vi "H-MEDI HardWareCtl.vi"() -> ()   [LabVIEW 2023]
uses:
  Controller/commonBtn.ctl
  <vilib>/Platform/TimedLoop/XDataNode/timing_clust.ctl
  <vilib>/Platform/TimedLoop/XDataNode/nitl_modes.ctl
  <vilib>/Platform/TimedLoop/XDataNode/wakeup.ctl
  <vilib>/Utility/miscctls.llb/LVPointTypeDef.ctl
  globalValue.vi
  <vilib>/Platform/TimedLoop/XDataNode/XDataNode.xnode
  <vilib>/Platform/TimedLoop/XDataNode/XDNodeRunTimeDep.lvlib
panel:
  in  "정지":bool
  out "userHeight":string
  out "userAge":string
  out "userGender":string
  in  "보행정보Menu":bool
  out "Tab":enum32{"1", "2", "3", "4", "Set"}(tab)
  out "rightIndicator#1-1":dbl
  out "leftIndicator#1-1":dbl
  out "leftIndicator#2-1":dbl
  out "rightIndicator#2-1":dbl
  out "leftIndicator#2-2":dbl
  out "rightIndicator#2-2":dbl
  out "leftIndicator#3-1":dbl
  out "rightIndicator#3-1":dbl
  out "leftIndicator#3-2":dbl
  out "rightIndicator#3-2":dbl
  out "leftIndicator#3-3":dbl
  out "rightIndicator#3-3":dbl
  out "leftIndicator#4-1":dbl
  out "rightIndicator#4-1":dbl
  out "leftIndicator#4-2":dbl
  out "rightIndicator#4-2":dbl
  out "leftIndicator#4-3":dbl
  out "rightIndicator#4-3":dbl
  out "leftIndicator#4-4":dbl
  out "rightIndicator#4-4":dbl
  in  "monitoringDataSet":bool
  in  "보행 지표":T1
  in  "Home":bool
  out "userInfo":string="000cm /  00kg"
  out "roleInfo":string
  out "R_GCP":dbl(slide) scale=0.0..100.0
  out "L_GCP":dbl(slide) scale=0.0..100.0
  out "R_THIGH":sgl
  out "L_Force":sgl
  out "R_Force":sgl
  out "Ref_L":sgl
  out "Ref_R":sgl
  out "Velocity_L":sgl
  out "Pos_L":sgl
  out "Velocity_R":sgl
  out "Pos_R":sgl
  out "L_THIGH":sgl
  in  "System Off":bool
  in  "start":bool
  in  "stop":bool
  in  "tabButton":enum32{"기본설정", "세부 설정", "메모"}(radio)
  out "Time":dbl format="%<%H:%M:%S>t"
  out "담당자 이름":string caption="담당자:"
  out "userName":string
  in  "Error":bool
  out "Battery":u16(ring)
  in  "Bluetooth":bool
  in  "사이드 탭":enum32{"Total", "Right", "Left", "메모"}(tab)
  in  "totalUserContolForce":T2
  in  "totalUserContolRelease":T2
  in  "totalUserContolPeak":T2
  in  "totalUserContolOnset":T2
  in  "leftUserContolRelease":T2
  in  "leftUserContolOnset":T2
  in  "leftUserContolPeak":T2
  in  "leftUserContolForce":T2
  in  "rightUserContolPeak":T2
  in  "rightUserContolOnset":T2
  in  "rightUserContolRelease":T2
  in  "rightUserContolForce":T2
  in  "메모 컨트롤":string="메모를 입력하세요."
  in  "메모 설정":bool
  out "Exit?":bool=TRUE
  in  "Connect":bool
  in  "Setting Value":T3={"Output High"=40.0, "Output Low"=-40.0, "Vel_FindBase"=5.0, "Ref.Load_FindBase"=5.0, "Force Peak"=0.0, "L_기준값"=81.0, "L_검출값"=103.0, "L_End%"=39.0, "L_Peak%"=25.0, "L_Onset%"=0.0, "L_Pos"=0.0, "L_Offset"=0.0, "R_기준값"=81.0, "R_검출값"=103.0, "R_End%"=39.0, "R_Peak%"=25.0, "R_Onset%"=0.0, "R_Pos"=0.0, "R_Offset"=0.0}
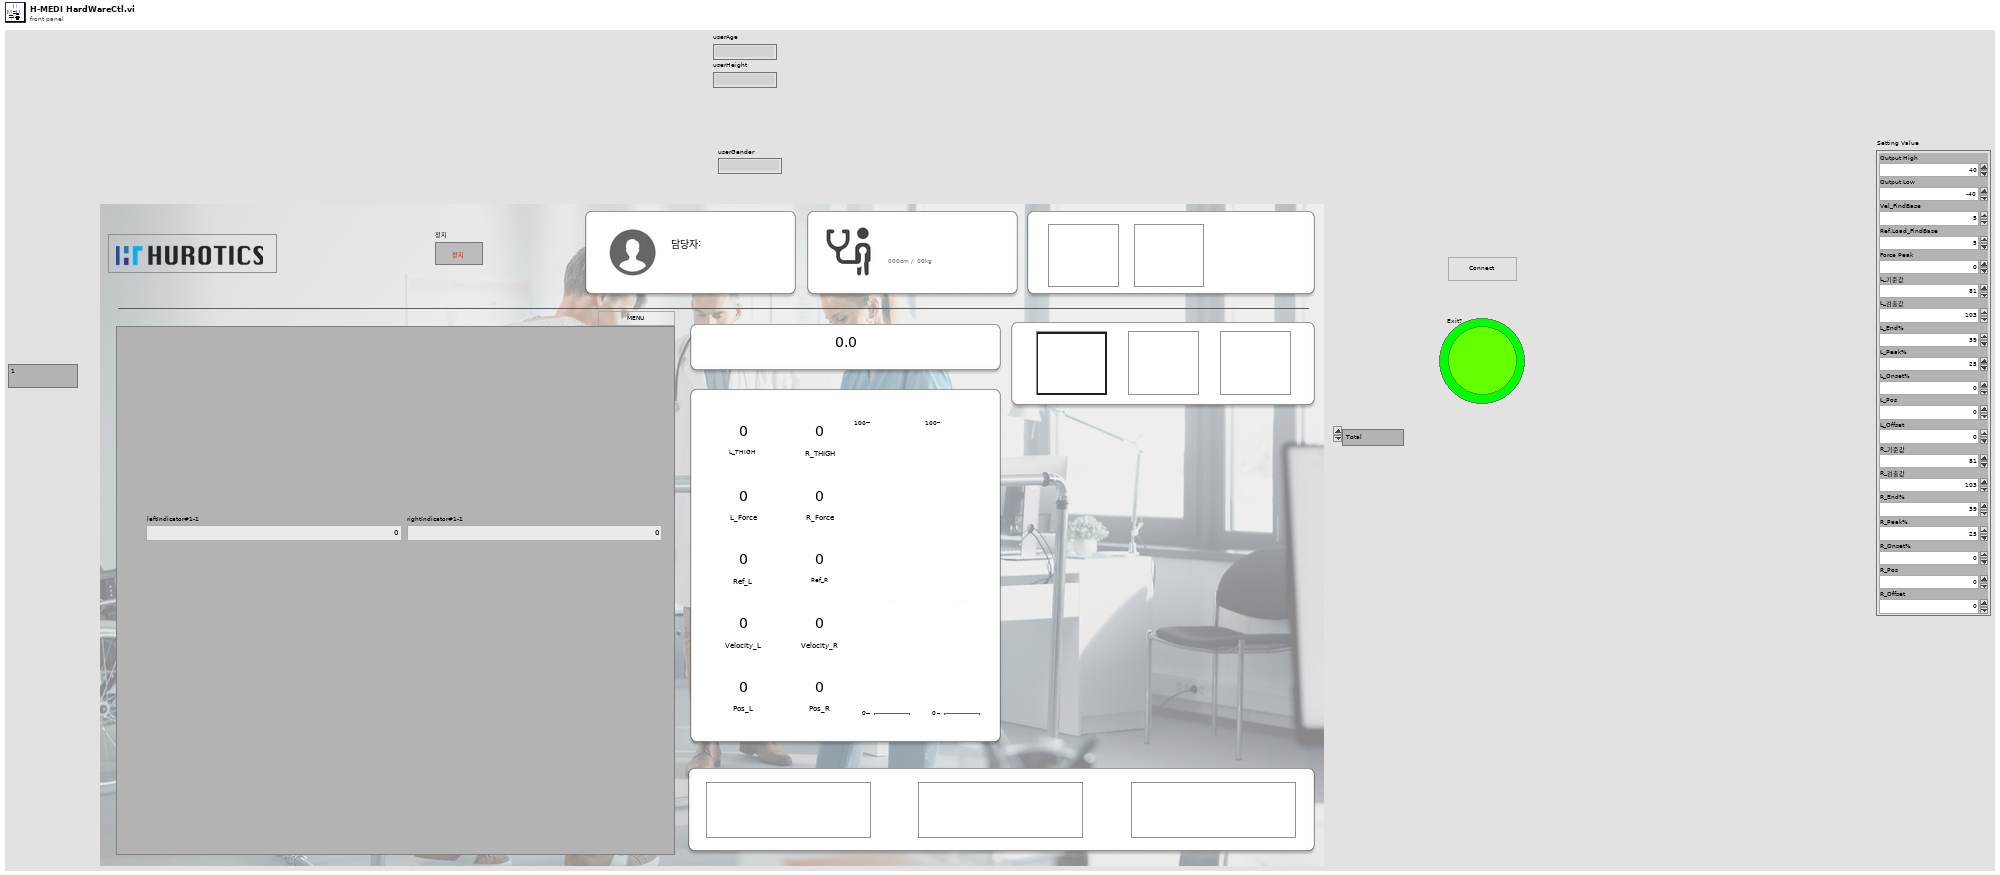
[diagram p1: front panel]
types:
  T1 = cluster{"고관절 각도":bool, "보행 속도":bool, "보행 거리":bool, "분당 걸음 수":bool, "보폭":bool, "Flexion / Extention":bool, "Range of Motion (ROM)":bool, "현 신체 균형":bool, "좌측만 보기":bool, "우측만 보기":bool}
  T2 = typedef "commonBtn.ctl" = i32
  T3 = cluster{"Output High":sgl, "Output Low":sgl, "Vel_FindBase":sgl, "Ref.Load_FindBase":sgl, "Force Peak":sgl, "L_기준값":sgl, "L_검출값":sgl, "L_End%":sgl, "L_Peak%":sgl, "L_Onset%":sgl, "L_Pos":sgl, "L_Offset":sgl, "R_기준값":sgl, "R_검출값":sgl, "R_End%":sgl, "R_Peak%":sgl, "R_Onset%":sgl, "R_Pos":sgl, "R_Offset":sgl}
  T4 = typedef "LVPointTypeDef.ctl" = cluster{"Horizontal":i16, "Vertical":i16}
  T5 = enum16{"connection", "create", "getReadList", "getRead", "getCount", "update", "delete", "close"}
  T6 = cluster{"baud rate (9600)":u32, "flow control (0:none)":u16, "VISA resource name 2":refnum<visa-resource-name>, "termination char\n(0xA = '\\n' = LF) ":u8, "data bits (8)":u16, "parity (0:none)":enum16{"None", "Odd", "Even", "Mark", "Space"}, "timeout (10sec)":u32, "Enable Termination\nChar (T)":bool, "stop bits (10: 1 bit)":u16}
  T7 = typedef "XDNodeRunTimeDep.lvlib/timing_clust.ctl" = cluster{"Expected End [f-1]":u64, "Actual End [f-1]":u64, "Finished Late? [f-1]":bool, "Expected End [i-1]":u64, "Actual End [i-1]":u64, "Finished Late? [i-1]":bool, "Expected Start [i]":u64, "Actual Start [i]":u64, "Expected Start [f]":u64, "Actual Start [f]":u64, "Source Name":string, "Structure Name":string, "Period":i64, "Deadline":i64, "Offset":i64, "Start":i64, "Priority":i32, "Timeout":i32, "Mode":T8, "Wakeup Reason":T9, "Error":errorcluster, "Source Type":string, "Secondary Source Type":string, "Global End Time":u64, "Global Start Time":u64, "Frame Duration":u64, "Iteration Duration":u64, "Assigned CPU":i32, "I/O Scan Engine Mode":u32}
  T8 = typedef "XDNodeRunTimeDep.lvlib/nitl_modes.ctl" = enum32{"No Change", "Process missed periods, maintain original phase", "Discard missed periods, maintain original phase", "Process missed periods, ignore original phase", "Discard missed periods, ignore original phase"}
  T9 = typedef "XDNodeRunTimeDep.lvlib/wakeup.ctl" = enum32{"Normal", "Aborted", "Asynchronous wakeup", "Timing source error", "Timed loop error", "Timeout"}
  T10 = enum16{"Open", "Write Only", "Read Only", "Write&Read", "Close"}
  T11 = enum16{"Init", "LogIn", "SignUpView", "Home", "Management_patientList", "Management_patientTrashtList", "Management_patientCreate", "Management_patientUpdate", "Management_patientTraining", "Management_patientTrainingDetail", "H-MEDI PatientList", "H-MEDI HardwareCtl", "Adjust", "FineTuning", "UserList", "UserDetail", "Exit"}
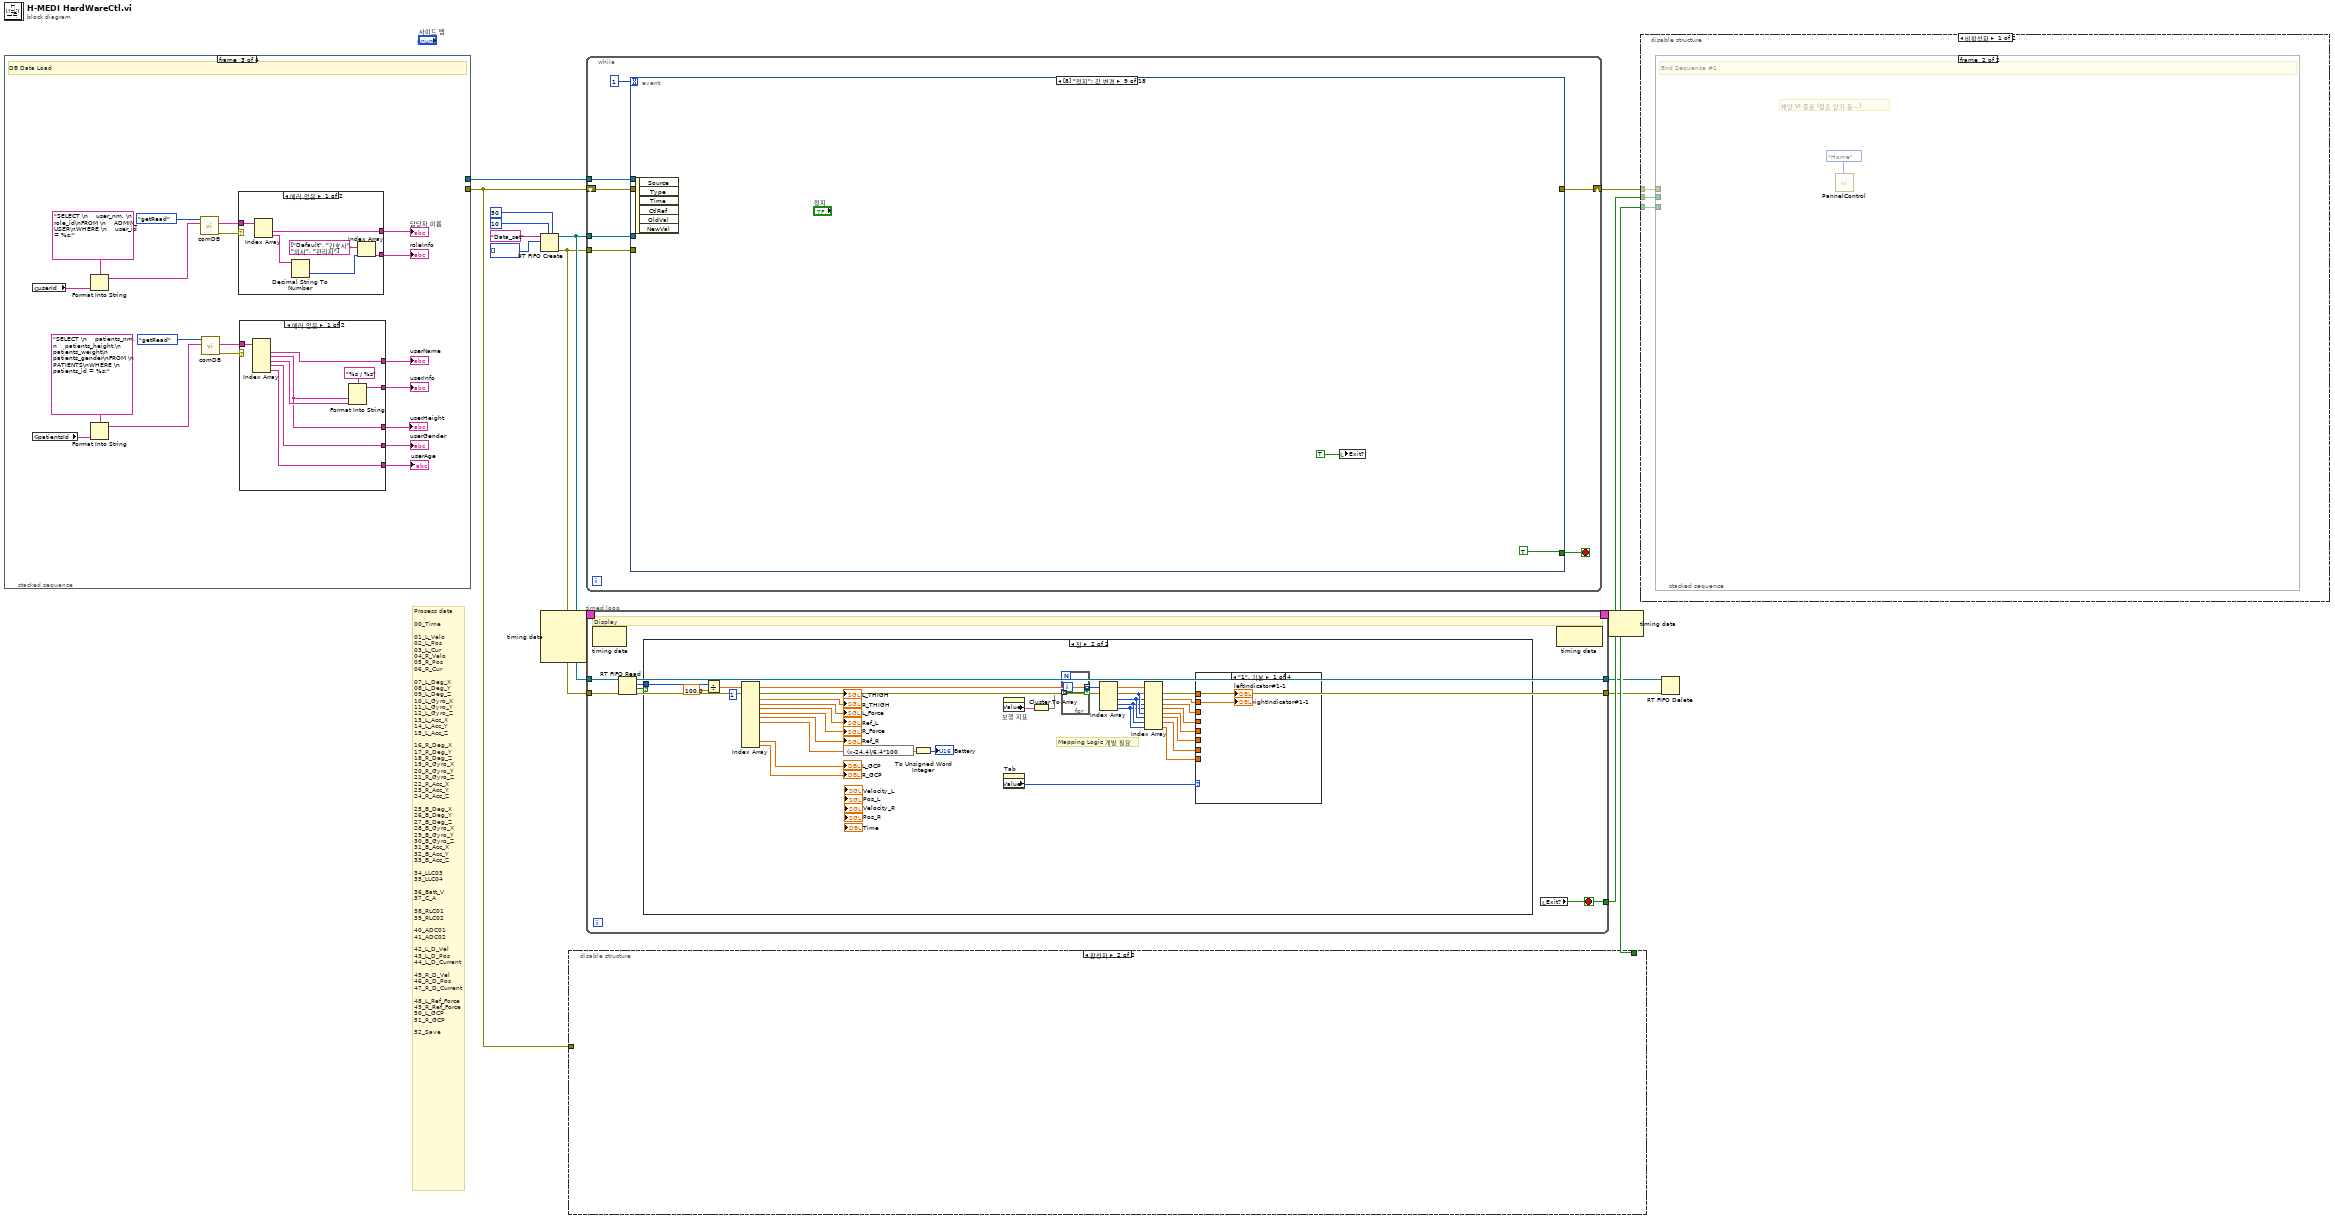
[diagram p0: block diagram]
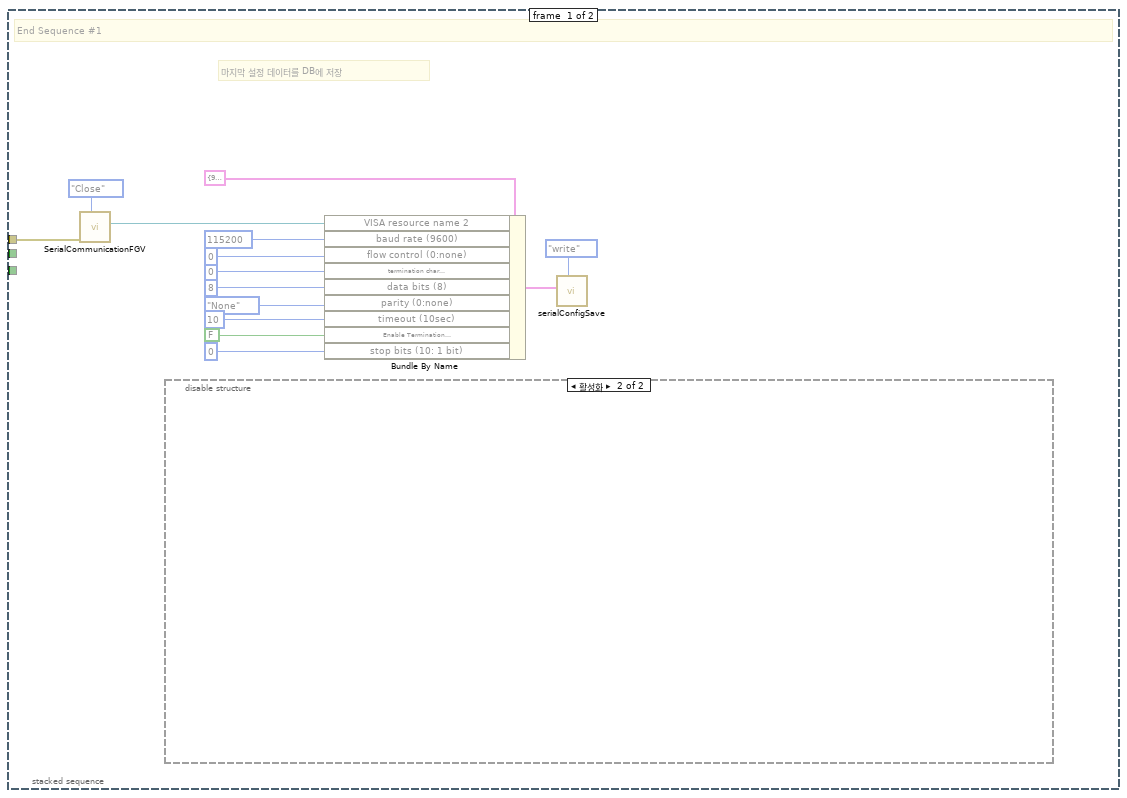
[diagram p2: hidden frame]
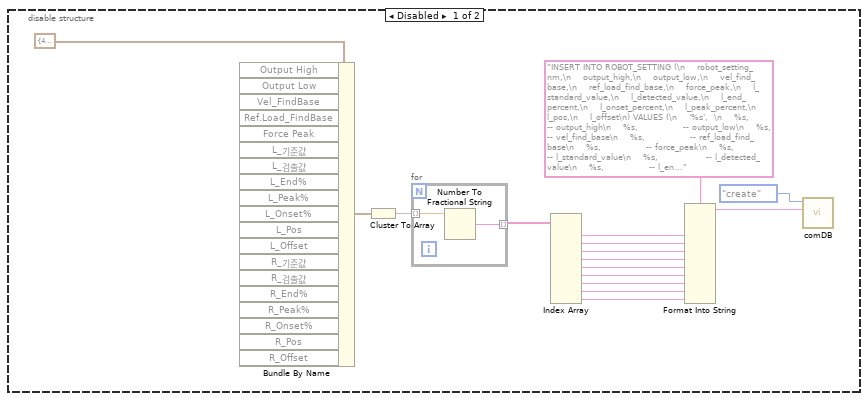
[diagram p3: hidden frame]
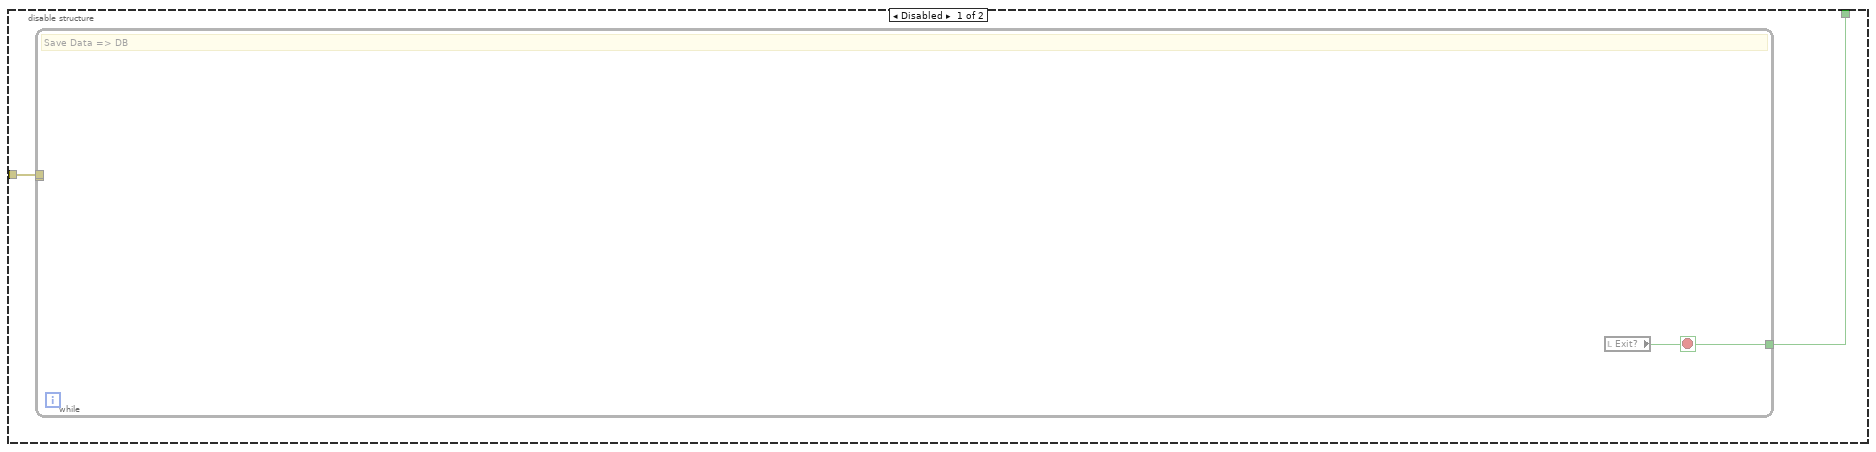
[diagram p5: hidden frame]
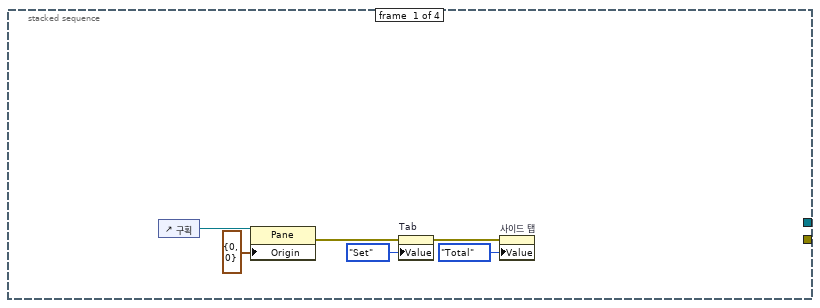
[diagram p6: hidden frame]
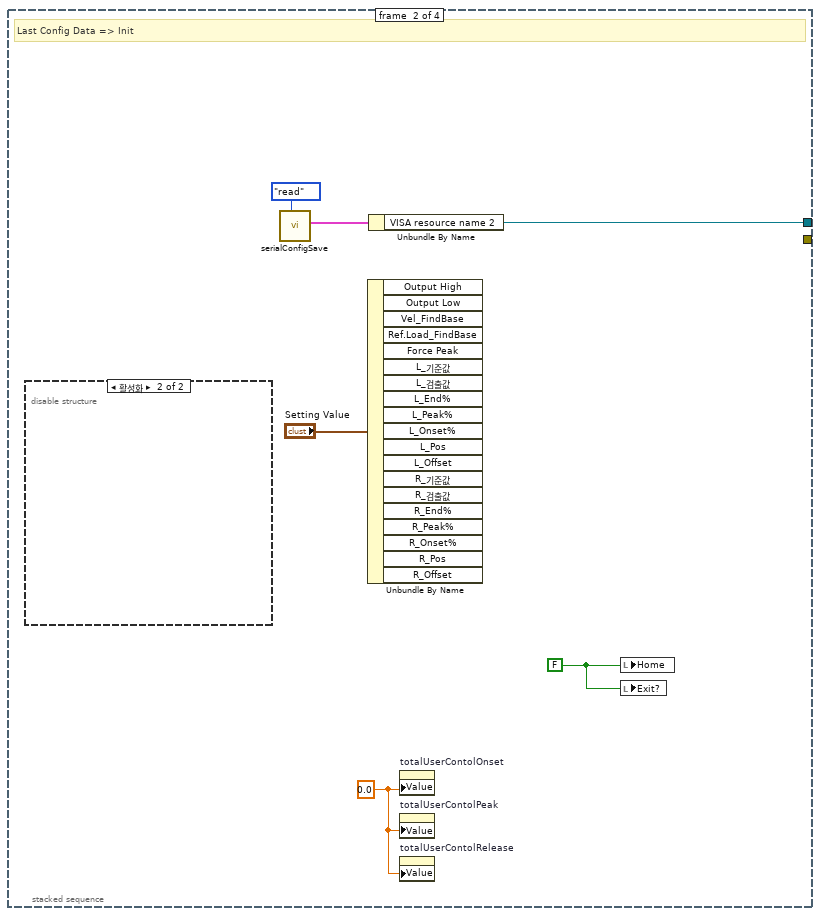
[diagram p7: hidden frame]
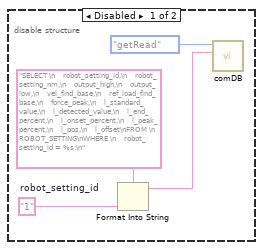
[diagram p8: hidden frame]
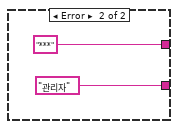
[diagram p9: hidden frame]
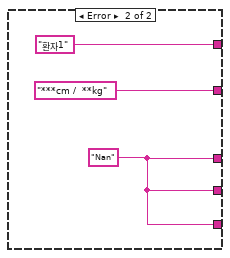
[diagram p10: hidden frame]
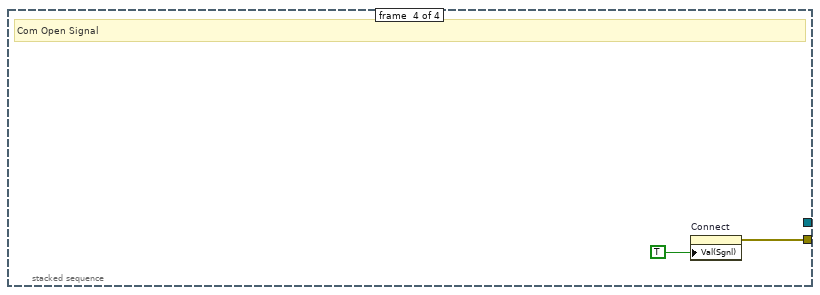
[diagram p11: hidden frame]
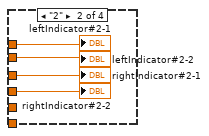
[diagram p13: hidden frame]
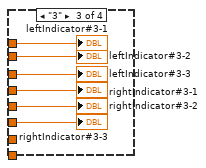
[diagram p14: hidden frame]
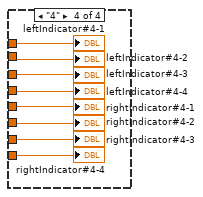
[diagram p15: hidden frame]
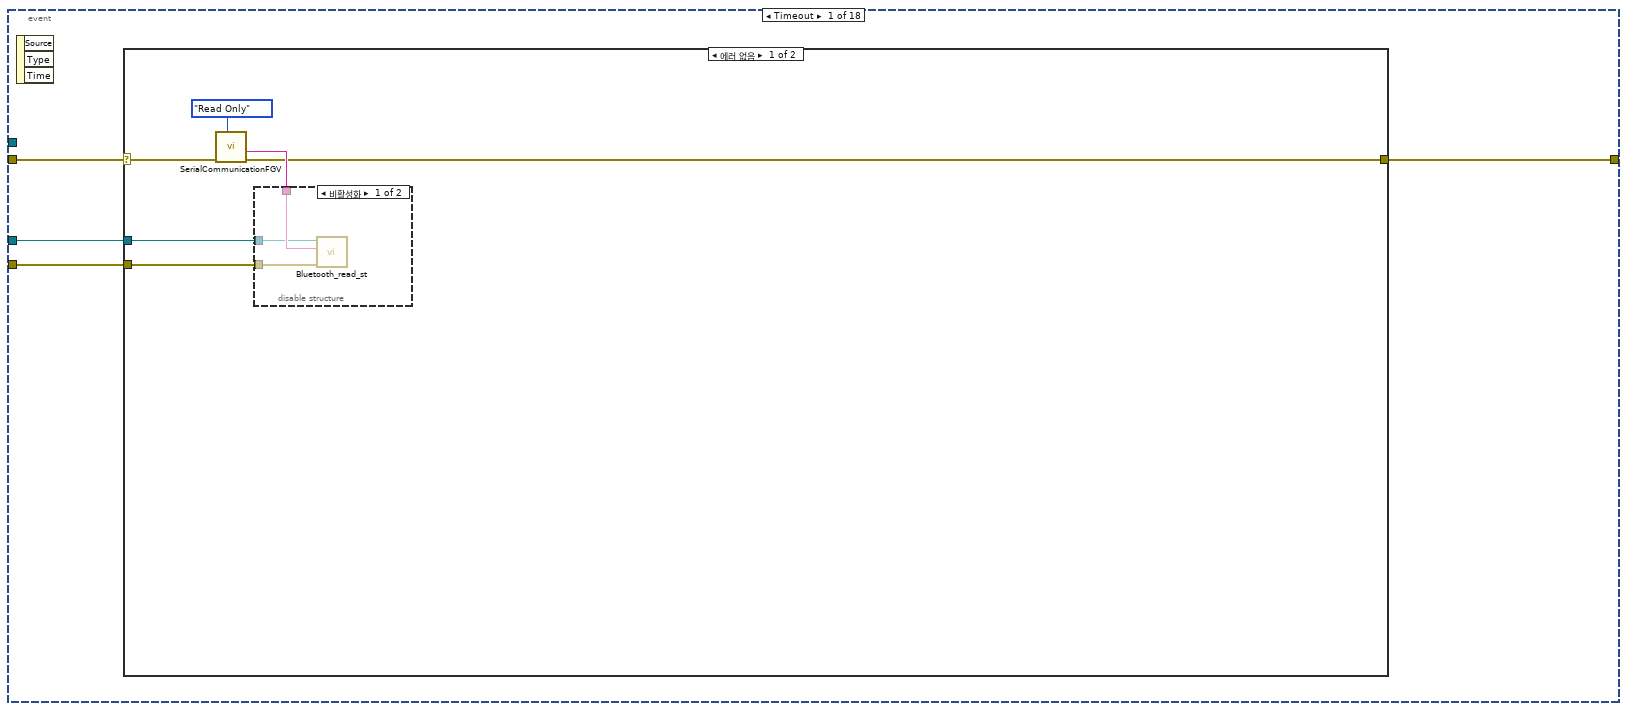
[diagram p16: hidden frame]
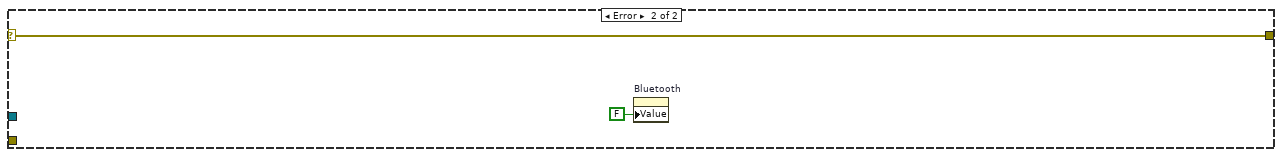
[diagram p18: hidden frame]
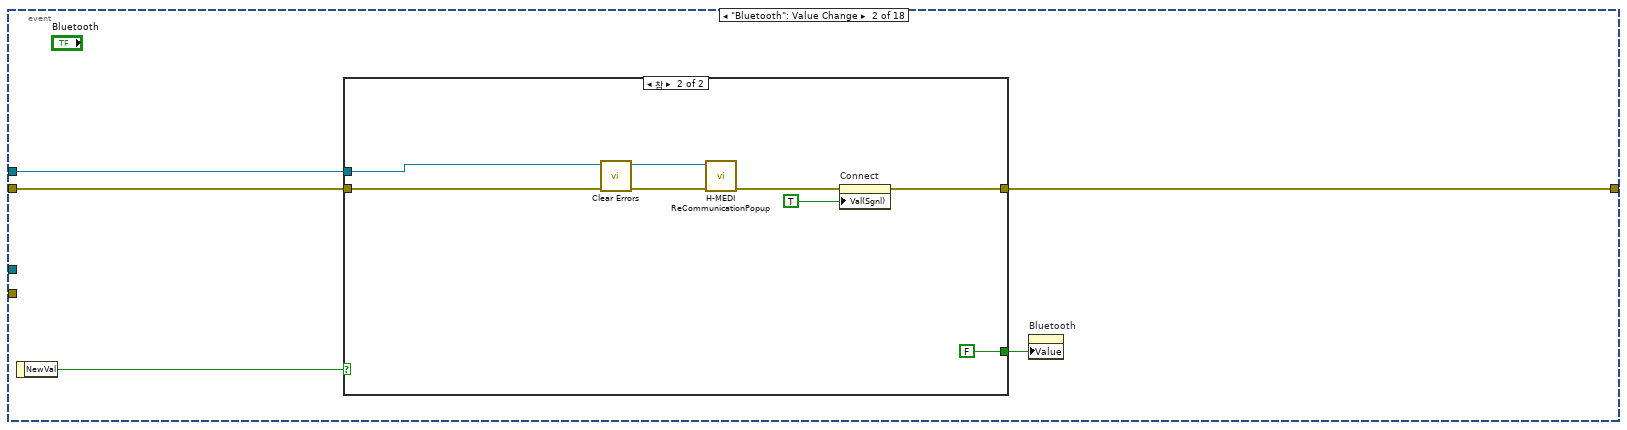
[diagram p19: hidden frame]
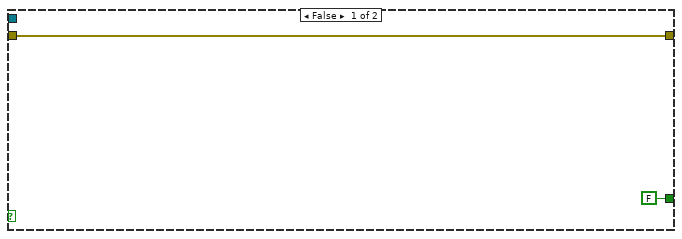
[diagram p20: hidden frame]
diagram:
  # "Prosess data\n\n00_Time\n\n01_L_Velo\n02_L_Pos\n03_L_Cur\n04_R_Velo\n05_R_Pos\n06_R_Cur\n\n07_L_Deg_X\n08_L_Deg_Y\n09_L_Deg_Z\n10_L_Gyro_X\n11_L_Gyro_Y\n12_L_Gyro_Z\n13_L_Acc_X\n14_L_Acc_Y\n15_L_Acc_Z\n\n16_R_Deg_X\n17_R_Deg_Y\n18_R_Deg_Z\n19_R_Gyro_X\n20_R_Gyro_Y\n21_R_Gyro_Z\n22_R_Acc_X\n23_R_Acc_Y\n24_R_Acc_Z\n\n25_B_Deg_X\n26_B_Deg_Y\n27_B_Deg_Z\n28_B_Gyro_X\n29_B_Gyro_Y\n30_B_Gyro_Z\n31_B_Acc_X\n32_B_Acc_Y\n33_B_Acc_Z\n\n34_LLC03\n35_LLC04\n\n36_Batt_V\n37_C_A\n\n38_RLC01\n39_RLC02\n\n40_ADC01\n41_ADC02\n\n42_L_D_Vel\n43_L_D_Pos\n44_L_D_Current\n\n45_R_D_Vel\n46_R_D_Pos\n47_R_D_Current\n\n48_L_Ref_Force\n49_R_Ref_Force\n50_L_GCP\n51_R_GCP\n\n52_Save"
  n1 = stacked-sequence {
    tunnel: [_ _ _ w70] -> w4
    tunnel: [_ w26 _ _] -> w10
    frame #0 {
      n2 = control-ref of="구획"() -> (w21:refnum<vi>)
      n3 = property class="Pane"(reference=w21, "Origin"=T4 {"Horizontal"=0, "Vertical"=0} ("원점")) -> (error out=w19:errorcluster)  [unwired: 1 in, 1 out]
      n4 = property on="Tab" class="TabCtl (엄격한)"(error in=w19, "Value"=enum32{"1", "2", "3", "4", "Set"}."Set" ("Tab")) -> (error out=w17:errorcluster)  [unwired: 1 in, 1 out]
      n5 = property on="사이드 탭" class="TabCtl (엄격한)"(error in=w17, "Value"=enum32{"Total", "Right", "Left", "메모"}."Total" ("사이드 탭")) -> ()  [unwired: 1 in, 2 out]
    }
    frame #1 {
      w25 = 0.0 ("Onset")
      w24 = FALSE ("정지")
      # "Last Config Data => Init"
      n6 = disable-structure shown="활성화" {
        frame Disabled {
          w29 = "1"  # robot_setting_id
          n7 = Format Into String(format string="SELECT \n    robot_setting_id,\n    robot_setting_nm,\n    output_high,\n    output_low,\n    vel_find_base,\n    ref_load_find_base,\n    force_peak,\n    l_standard_value,\n    l_detected_value,\n    l_end_percent,\n    l_onset_percent,\n    l_peak_percent,\n    l_pos,\n    l_offset\nFROM \n    ROBOT_SETTING\nWHERE \n    robot_setting_id = %s;\n", w29) -> (resulting string=w28:string)  [unwired: 2 in, 1 out]
          n8 = call "comDB.vi"("Query"=w28, "State"=T5."getRead") -> ()  [unwired: 5 in, 4 out]
        }
        frame Enabled {
        }
      }
      n9 = call "serialConfigSave.vi"("Ctl"=enum16{"read", "write"}."read") -> ("Reurn"=w22:T6)  [unwired: 10 in]
      n10 = Unbundle By Name("Setting Value") -> ()  [unwired: 19 out]
      n11 = Unbundle By Name(w22) -> ("VISA resource name 2"=w26:refnum<visa-resource-name>)
      n12 = property on="totalUserContolOnset" class="DigNum (엄격한)"("Value"=w25) -> ()  [unwired: 2 in, 2 out]
      n13 = property on="totalUserContolPeak" class="DigNum (엄격한)"("Value"=w25) -> ()  [unwired: 2 in, 2 out]
      n14 = property on="totalUserContolRelease" class="DigNum (엄격한)"("Value"=w25) -> ()  [unwired: 2 in, 2 out]
      n15 = local write "Home"(w24) -> ()
      n16 = local write "Exit?"(w24) -> ()
    }
    frame #2 {
      # "DB Data Load"
      n17 = global read "globalValue.vi" "userId"() -> (w40:string)
      n18 = global read "globalValue.vi" "patientsId"() -> (w43:string)
      n19 = Format Into String(format string="SELECT \n    user_nm, \n    role_id\nFROM \n    ADMIN_USER\nWHERE \n    user_id = %s;", w40) -> (resulting string=w39:string)  [unwired: 2 in, 1 out]
      n20 = Format Into String(format string="SELECT \n    patients_nm, \n    patients_height,\n    patients_weight\n    patients_gender\nFROM \n    PATIENTS\nWHERE \n    patients_id = %s;", w43) -> (resulting string=w46:string)  [unwired: 2 in, 1 out]
      n21 = call "comDB.vi"("Query"=w39, "State"=T5."getRead") -> ("error out"=w38:errorcluster, "result1DArray"=w35:string[])  [unwired: 5 in, 2 out]
      n22 = call "comDB.vi"("Query"=w46, "State"=T5."getRead") -> ("error out"=w45:errorcluster, "result1DArray"=w44:string[])  [unwired: 5 in, 2 out]
      n23 = case shown="에러 없음" w38 {
        tunnel: [w55 "***" ("담당자 이름")] -> w37
        tunnel: [w52 "관리자" ("roleInfo")] -> w36
        tunnel: w35 -> [w56 _]
        frame No Error {
          n24 = Index Array(array=w56) -> (element #1=w55:string, element #2=w54:string)  [unwired: 2 in]
          n25 = Decimal String To Number(string=w54) -> (number=w51:i32)  [unwired: 2 in, 1 out]
          n26 = Index Array(array=string[] ["Default", "간호사", "의사", "관리자"], index=w51) -> (element=w52:string)
        }
        frame Error {
        }
      }
      "담당자 이름" <- w37
      "roleInfo" <- w36
      n27 = case shown="에러 없음" w45 {
        tunnel: [w64 "환자1" ("환자이름")] -> w50
        tunnel: [w62 "***cm /  **kg" ("userInfo")] -> w49
        tunnel: w44 -> [w66 _]
        tunnel: [w61 w67] -> w34
        tunnel: [w60 w67] -> w33
        tunnel: [w59 w67] -> w32
        frame No Error {
          n28 = Index Array(array=w66) -> (element #1=w64:string, element #2=w59:string, element #3=w63:string, element #4=w61:string, element #5=w60:string)  [unwired: 5 in]
          n29 = Format Into String(format string="%s / %s" ("포맷 문자열"), w59, w63) -> (resulting string=w62:string)  [unwired: 2 in, 1 out]
        }
        frame Error {
          w67 = "Nan" ("Text")
        }
      }
      "userName" <- w50
      "userInfo" <- w49
      "userGender" <- w34
      "userAge" <- w33
      "userHeight" <- w32
    }
    frame #3 {
      # "Com Open Signal"
      n30 = property on="Connect" class="Bool (엄격한)"("Val(Sgnl)"=TRUE ("값(신호)")) -> (error out=w70:errorcluster)  [unwired: 2 in, 1 out]
    }
  }
  n31 = RT FIFO Create(0:"Data_set" ("이름(이름없음)"), 1:i32[] [], 4:u32 10 ("크기(10)"), 6:u32 50 ("배열의 원소(1)")) -> (8:w5:refnum<k33>, 11:w3:errorcluster)  [unwired: 4 in, 1 out]
  n32 = node-c288() -> (w15:T7)  [unwired: 4 in]
  n33 = disable-structure shown="활성화" {
    disable-tunnel: w4 -> [w73 _]
    disable-tunnel: [w72 _] -> w11
    frame Disabled {
      n34 = while {
        tunnel: [w75] -> _
        tunnel: w73 -> [w75]
        tunnel: [w74] -> w72
        stop <- w74 stop-if-true
        # "Save Data => DB"
        n35 = local read "Exit?"() -> (w74:bool)
      }
    }
    frame Enabled {
    }
  }
  n36 = while {
    shift-right: [w79] -> w13
    shift-left: w4 -> [w80]
    tunnel: w10 -> [w78]
    tunnel: w5 -> [w77]
    tunnel: w3 -> [w76]
    stop <- w82 stop-if-true
    n37 = event shown="[8] \"정지\": 값 변경" {
      selector: _ -> [_ _ _ _ _ _ _ _ _ _ _ _ _ _ _ _ _ _]
      dyn-events: _ -> [_ _ _ _ _ _ _ _ _ _ _ _ _ _ _ _ _ _]
      timeout: 1 -> [_ _ _ _ _ _ _ _ _ _ _ _ _ _ _ _ _ _]
      tunnel: [_ _ _ _ _ _ _ _ TRUE _ _ _ _ _ _ _ w253 w256] -> w82
      tunnel: w78 -> [_ w100 w114 _ _ _ _ _ _ _ _ _ _ _ _ _ _ _]
      tunnel: w80 -> [w86 w102 w112 w142 w151 w161 w171 w179 _ w189 w198 w216 w232 w245 w247 w248 w254 w255]
      tunnel: [w83 w101 w113 w142 w151 w161 w170 w178 _ w188 w195 w211 w231 w243 w247 w248 w254 w255] -> w79
      tunnel: w77 -> [w85 _ _ _ _ _ _ _ _ _ _ _ _ _ _ _ _ _]
      tunnel: w76 -> [w84 _ _ _ _ _ _ _ _ _ _ _ _ _ _ _ _ _]
      event Timeout {
        n38 = event-data() -> ()  [unwired: 1 in, 3 out]
        n39 = case shown="에러 없음" w86 {
          selector: w86 -> [w91 w96]
          tunnel: w85 -> [w89 _]
          tunnel: w84 -> [w88 _]
          tunnel: [w87 w96] -> w83
          frame No Error {
            n40 = call "SerialCommunicationFGV.vi"("ctl"=T10."Read Only", "errorIn"=w91) -> ("errorOut"=w87:errorcluster, "bufferRead"=w90:string)  [unwired: 7 in, 1 out]
            n41 = disable-structure shown="비활성화" {
              disable-tunnel: w90 -> [w95 _]
              disable-tunnel: w89 -> [w94 _]
              disable-tunnel: w88 -> [w93 _]
              frame Disabled {
                n42 = call "Bluetooth_read_st.vi"("Err_IN"=w93, "read buffer"=w95, "Data_set"=w94) -> ()  [unwired: 5 in, 4 out]
              }
              frame Enabled {
              }
            }
          }
          frame Error {
            n43 = property on="Bluetooth" class="Bool (엄격한)"("Value"=FALSE ("Bluetooth")) -> ()  [unwired: 2 in, 2 out]
          }
        }
      }
      event "Bluetooth": Value Change {
        n44 = event-data() -> ("NewVal"=w99:bool)  [unwired: 1 in]
        n45 = case shown="참" w99 {
          tunnel: w102 -> [w103 w111]
          tunnel: [w103 w105] -> w101
          tunnel: w100 -> [_ w109]
          tunnel: [FALSE FALSE] -> w98
          frame False {
          }
          frame True {
            n46 = call <vilib>:"Clear Errors.vi"("error in (no error)"=w111) -> ("error out"=w110:errorcluster)  [unwired: 5 in, 1 out]
            n47 = call "H-MEDI ReCommunicationPopup.vi"("에러 입력(에러 없음)"=w110, "inputResourceName"=w109) -> ("error out"=w107:errorcluster)  [unwired: 8 in, 1 out]
            n48 = property on="Connect" class="Bool (엄격한)"(error in=w107, "Val(Sgnl)"=TRUE ("값(신호)")) -> (error out=w105:errorcluster)  [unwired: 1 in, 1 out]
          }
        }
        n49 = property on="Bluetooth" class="Bool (엄격한)"("Value"=w98) -> ()  [unwired: 2 in, 2 out]
      }
      event "Connect": Value Change {
        n50 = event-data() -> ("NewVal"=w116:bool)  [unwired: 1 in]
        n51 = case shown="참" w116 {
          tunnel: [FALSE FALSE] -> w115
          tunnel: w114 -> [_ w139]
          tunnel: [w117 w130] -> w113
          tunnel: w112 -> [w117 w138]
          frame False {
          }
          frame True {
            n52 = property on="userAge" class="Str"() -> ("Value"=w128:string)  [unwired: 2 in, 2 out]
            n53 = property on="userHeight" class="Str"() -> ("Value"=w126:string)  [unwired: 2 in, 2 out]
            n54 = property on="userGender" class="Str"() -> ("Value"=w122:string)  [unwired: 2 in, 2 out]
            n55 = Equal?(x=w122, y="Male") -> (x = y?=w120:bool)
            n56 = Decimal String To Number(string=w128, default (0L)=0.0) -> (number=w127:dbl)  [unwired: 1 in, 1 out]
            n57 = Decimal String To Number(string=w126, default (0L)=0.0) -> (number=w125:dbl)  [unwired: 1 in, 1 out]
            n58 = Boolean To (0,1)(Boolean=w120) -> (0, 1=w119:i16)
            n59 = call "SerialCommunicationFGV.vi"("ctl"=T10."Open", "errorIn"=w138, "visaResourceNameIn"=w139) -> ("errorOut"=w134:errorcluster)  [unwired: 6 in, 2 out]
            n60 = call "Time SET.vi"() -> ("배열"=w136:i32[])  [unwired: 10 in, 1 out]
            n61 = call "Gender_Age_Hight.vi"("Gender"=w119, "height"=w125, "age"=w127) -> ("Dataset"=w133:i32[])  [unwired: 8 in]
            n62 = Type Cast(x=w136) -> (*(type *) &x=w135:string)  [unwired: 1 in]
            n63 = Type Cast(x=w133) -> (*(type *) &x=w132:string)  [unwired: 1 in]
            n64 = call "SerialCommunicationFGV.vi"("ctl"=T10."Write&Read", "errorIn"=w134, "bufferWrite"=w135) -> ("errorOut"=w131:errorcluster)  [unwired: 6 in, 2 out]
            n65 = call "SerialCommunicationFGV.vi"("ctl"=T10."Write&Read", "errorIn"=w131, "bufferWrite"=w132) -> ("errorOut"=w130:errorcluster)  [unwired: 6 in, 2 out]
          }
        }
        n66 = property on="Connect" class="Bool (엄격한)"("Value"=w115) -> ()  [unwired: 2 in, 2 out]
      }
      event "보행정보Menu": Value Change {
        n67 = event-data() -> ()  [unwired: 1 in, 6 out]
        n68 = property on="Tab" class="TabCtl (엄격한)"("Value"=enum32{"1", "2", "3", "4", "Set"}."Set" ("Tab")) -> ()  [unwired: 2 in, 2 out]
      }
      event "보행 지표": Value Change {
        n69 = event-data() -> ("OldVal"=w144:T1)  [unwired: 1 in, 5 out]
        n70 = Cluster To Array(cluster="보행 지표") -> (array=w149:bool[])
        n71 = for {
          tunnel: w149 -> [w156] mode=indexing
          tunnel: [w156] -> w150 mode=indexing if=w156
        }
        n72 = Array Size(array=w150) -> (size(s)=w147:i32)
        n73 = Greater Or Equal?(x=w147, y=5) -> (x >= y?=w145:bool)
        n74 = case shown="참" w145 {
          tunnel: w144 -> [_ w153]
          frame False {
          }
          frame True {
            n75 = One Button Dialog(message="보형 지표는  최대 4개까지 선택 가능합니다." ("메시지")) -> (true=w152:bool)  [unwired: 1 in]
            n76 = flat-sequence {
              tunnel: w153 -> [w155]
              tunnel: w152 -> [_]
              frame #0 {
                n77 = property on="보행 지표" class="Clust (엄격한)"("Value"=w155) -> ()  [unwired: 2 in, 2 out]
              }
            }
          }
        }
      }
      event "monitoringDataSet": Value Change {
        n78 = event-data() -> ()  [unwired: 1 in, 6 out]
        n79 = property on="보행 지표" class="Clust (엄격한)"() -> ("Value"=w157:T1)  [unwired: 2 in, 2 out]
        n80 = Cluster To Array(cluster=w157) -> (array=w158:bool[])
        n81 = for {
          tunnel: w158 -> [w168] mode=indexing
          tunnel: [w168] -> w160 mode=indexing if=w168
        }
        n82 = Array Size(array=w160) -> (size(s)=w159:i32)
        n83 = case shown="1..4" w159 {
          selector: w159 -> [_ w165 _]
          frame 0 {
            n84 = One Button Dialog(message="데이터를 선택해주세요." ("메시지")) -> ()  [unwired: 1 in, 1 out]
          }
          frame 1..4 {
            n85 = Decrement(x=w165) -> (x-1=w164:i32)
            n86 = property on="Tab" class="TabCtl (엄격한)"() -> ("Value"=w166:enum32{"1", "2", "3", "4", "Set"})  [unwired: 2 in, 2 out]
            n87 = Type Cast(type=w166, x=w164) -> (*(type *) &x=→"Tab":enum32{"1", "2", "3", "4", "Set"})
          }
          frame 5, Default {
            n88 = One Button Dialog(message="보형 지표는  최대 4개까지 선택 가능합니다." ("메시지")) -> ()  [unwired: 1 in, 1 out]
          }
        }
      }
      event "start": Value Change {
        n89 = event-data() -> ("NewVal"=w169:bool)  [unwired: 1 in]
        n90 = case shown="참" w169 {
          tunnel: w171 -> [w172 w175]
          tunnel: [w172 w174] -> w170
          frame False {
            (unwired) FALSE
          }
          frame True {
            n91 = call "SerialCommunicationFGV.vi"("ctl"=T10."Write Only", "errorIn"=w175, "bufferWrite"="\u0000\u0000\u0000\u0002\u0000\u0000\u0000\u0001\u0000\u0000\u0000\u0001\u0000\u0000\u0000\u0001\u0000\u0000\u0000\u0000\u0000\u0000\u0000\u0000\u0000\u0000\u0000\u0000\u0000\u0000\u0000\u0000\u0000\u0000\u0000\u0000\u0000\u0000\u0000\u0000\u0000\u0000\u0000\u0000\u0000\u0000\u0000\u0001\u0000\u0000\u0000\u0003" ("*(타입 *) &x")) -> ("errorOut"=w174:errorcluster)  [unwired: 6 in, 2 out]
          }
        }
      }
      event "stop": Value Change {
        n92 = event-data() -> ("NewVal"=w177:bool)  [unwired: 1 in]
        n93 = case shown="참" w177 {
          tunnel: w179 -> [w180 w183]
          tunnel: [w180 w182] -> w178
          frame False {
            (unwired) FALSE
          }
          frame True {
            n94 = call "SerialCommunicationFGV.vi"("ctl"=T10."Write Only", "errorIn"=w183, "bufferWrite"="\u0000\u0000\u0000\u0002\u0000\u0000\u0000\u0001\u0000\u0000\u0000\u0001\u0000\u0000\u0000\u0000\u0000\u0000\u0000\u0000\u0000\u0000\u0000\u0000\u0000\u0000\u0000\u0000\u0000\u0000\u0000\u0000\u0000\u0000\u0000\u0000\u0000\u0000\u0000\u0000\u0000\u0000\u0000\u0000\u0000\u0000\u0000\u0000\u0000\u0000\u0000\u0003" ("*(타입 *) &x")) -> ("errorOut"=w182:errorcluster)  [unwired: 6 in, 2 out]
          }
        }
      }
      event "정지": Value Change {
        n95 = event-data() -> ()  [unwired: 1 in, 6 out]
        n96 = local write "Exit?"(TRUE ("Exit?")) -> ()
      }
      event "System Off": Value Change {
        n97 = event-data() -> ("NewVal"=w187:bool)  [unwired: 1 in]
        n98 = case shown="참" w187 {
          tunnel: w189 -> [w190 w193]
          tunnel: [w190 w192] -> w188
          frame False {
            (unwired) FALSE
          }
          frame True {
            n99 = call "SerialCommunicationFGV.vi"("ctl"=T10."Write Only", "errorIn"=w193, "bufferWrite"="\u0000\u0000\u0000\u0002\u0000\u0000\u0000\u0001\u0000\u0000\u0000\u0002\u0000\u0000\u0000\u0000\u0000\u0000\u0000\u0000\u0000\u0000\u0000\u0000\u0000\u0000\u0000\u0000\u0000\u0000\u0000\u0000\u0000\u0000\u0000\u0000\u0000\u0000\u0000\u0000\u0000\u0000\u0000\u0000\u0000\u0000\u0000\u0002\u0000\u0000\u0000\u0003" ("*(타입 *) &x")) -> ("errorOut"=w192:errorcluster)  [unwired: 6 in, 2 out]
          }
        }
      }
      event Value Change {
        w203 = 0 ("원소")
        n100 = event-data() -> ()  [unwired: 1 in, 6 out]
        n101 = Build Array("totalUserContolOnset", "totalUserContolPeak", "totalUserContolRelease", "totalUserContolForce", w203, w203, w203, w203) -> (w201:T2[])
        n102 = Add Array Elements(numeric array=w201) -> (sum=w200:T2)
        n103 = Build Array (concatenate)(2 ("원소"), 1 ("원소"), 4 ("원소"), w201, 3 ("원소"), w200) -> (w197:T2[])
        n104 = Type Cast(x=w197) -> (*(type *) &x=w196:string)  [unwired: 1 in]
        n105 = call "SerialCommunicationFGV.vi"("ctl"=T10."Write Only", "errorIn"=w198, "bufferWrite"=w196) -> ("errorOut"=w195:errorcluster)  [unwired: 6 in, 2 out]
      }
      event Value Change {
        w221 = 0 ("원소")
        n106 = event-data() -> ()  [unwired: 1 in, 6 out]
        n107 = Build Array("leftUserContolOnset", "leftUserContolPeak", "leftUserContolRelease", "leftUserContolForce", w221, w221, w221, w221) -> (w226:T2[])
        n108 = Add Array Elements(numeric array=w226) -> (sum=w225:T2)
        n109 = Build Array (concatenate)(2 ("원소"), 1 ("원소"), 2 ("원소"), w226, 3 ("원소"), w225) -> (w224:T2[])
        n110 = Type Cast(x=w224) -> (*(type *) &x=w223:string)  [unwired: 1 in]
        n111 = call "SerialCommunicationFGV.vi"("ctl"=T10."Write Only", "errorIn"=w216, "bufferWrite"=w223) -> ("errorOut"=w211:errorcluster)  [unwired: 6 in, 2 out]
      }
      event Value Change {
        w237 = 0 ("원소")
        n112 = event-data() -> ()  [unwired: 1 in, 6 out]
        n113 = Build Array("rightUserContolOnset", "rightUserContolPeak", "rightUserContolRelease", "rightUserContolForce", w237, w237, w237, w237) -> (w242:T2[])
        n114 = Add Array Elements(numeric array=w242) -> (sum=w241:T2)
        n115 = Build Array (concatenate)(2 ("원소"), 1 ("원소"), 3 ("원소"), w242, 3 ("원소"), w241) -> (w240:T2[])
        n116 = Type Cast(x=w240) -> (*(type *) &x=w239:string)  [unwired: 1 in]
        n117 = call "SerialCommunicationFGV.vi"("ctl"=T10."Write Only", "errorIn"=w232, "bufferWrite"=w239) -> ("errorOut"=w231:errorcluster)  [unwired: 6 in, 2 out]
      }
      event "Error": Value Change {
        n118 = event-data() -> ()  [unwired: 1 in, 6 out]
        n119 = call "H-MEDI Error Popup.vi"("error in (no error)"=w245) -> ("error out"=w244:errorcluster)  [unwired: 9 in, 1 out]
        n120 = property on="Error" class="Bool (엄격한)"(error in=w244, "Value"=FALSE ("Error")) -> (error out=w243:errorcluster)  [unwired: 1 in, 1 out]
      }
      event "메모 설정": Value Change {
        n121 = event-data() -> ()  [unwired: 1 in, 6 out]
      }
      event "tabButton": Value Change {
        n122 = event-data() -> ("NewVal"=w249:enum32{"기본설정", "세부 설정", "메모"})  [unwired: 1 in, 5 out]
        n123 = case shown="\"기본설정\", 기본" w249 {
          frame "기본설정", Default {
            n124 = local write "사이드 탭"(enum32{"Total", "Right", "Left", "메모"}."Total" ("사이드 탭")) -> ()
          }
          frame "세부 설정" {
            n125 = local write "사이드 탭"(enum32{"Total", "Right", "Left", "메모"}."Right" ("사이드 탭")) -> ()
          }
          frame "메모" {
            n126 = local write "사이드 탭"(enum32{"Total", "Right", "Left", "메모"}."메모" ("사이드 탭")) -> ()
          }
        }
      }
      event "Home": Value Change {
        w253 = TRUE
        n127 = event-data() -> ()  [unwired: 1 in, 6 out]
        n128 = local write "Exit?"(w253) -> ()
      }
      event Panel Close {
        w256 = TRUE
        n129 = event-data() -> ()  [unwired: 1 in, 4 out]
        "Exit?" <- w256
      }
    }
  }
  n130 = timed-loop {
    timing: w15 -> [_]
    timing-out: [_] -> w14
    tunnel: w3 -> [w261]
    tunnel: [w263] -> w12
    tunnel: w5 -> [w262]
    tunnel: [w257] -> w2
    tunnel: [w260] -> w1
    stop <- w263 stop-if-true
    # "Display"
    n131 = node-c288() -> ()  [unwired: 1 in, 1 out]
    n132 = RT FIFO Read(0:w262, 3:w261) -> (8:w260:refnum<k33>, 9:w258:i32[], 10:w259:bool, 11:w257:errorcluster)  [unwired: 2 in, 1 out]
    n133 = case shown="참" w259 {
      tunnel: w258 -> [_ w294]
      frame False {
      }
      frame True {
        # "Mapping Logic 개발 필요"
        n134 = Divide(x=w294, y=sgl 100.0) -> (x/y=w275:sgl[])
        n135 = Index Array(array=w275, index #1=1 ("인덱스")) -> (element #1=→"L_THIGH":sgl, element #2=→"R_THIGH":sgl, element #3=→"L_Force":sgl, element #4=→"Ref_L":sgl, element #5=→"R_Force":sgl, element #6=→"Ref_R":sgl, element #7=w281:sgl, element #11=→"L_GCP":sgl, element #12=→"R_GCP":sgl)  [unwired: 11 in, 3 out]
        n136 = expression code="(x-24.4)/6.4*100"(w281) -> (w289:sgl)
        n137 = To Unsigned Word Integer(number=w289) -> (unsigned 16bit integer=→"Battery":u16)
        n138 = property on="보행 지표" class="Clust (엄격한)"() -> ("Value"=w279:T1)  [unwired: 2 in, 2 out]
        n139 = property on="Tab" class="TabCtl (엄격한)"() -> ("Value"=w280:enum32{"1", "2", "3", "4", "Set"})  [unwired: 2 in, 2 out]
        n140 = Cluster To Array(cluster=w279) -> (array=w278:bool[])
        n141 = for {
          tunnel: w278 -> [w295] mode=indexing
          tunnel: [w296] -> w277 mode=indexing if=w295
          i -> [w296]
        }
        n142 = Index Array(array=w277) -> (element #1=w267:i32, element #2=w266:i32, element #3=w265:i32, element #4=w264:i32)  [unwired: 4 in]
        n143 = Index Array(array=w275, index #1=w267, index #2=w266, index #3=w265, index #4=w264, index #5=w267, index #6=w266, index #7=w265, index #8=w264) -> (element #1=w276:sgl, element #2=w274:sgl, element #3=w273:sgl, element #4=w272:sgl, element #5=w271:sgl, element #6=w270:sgl, element #7=w269:sgl, element #8=w268:sgl)
        n144 = case shown="\"1\", 기본" w280 {
          tunnel: w276 -> [w298 w302 w308 w316]
          tunnel: w274 -> [w297 w301 w307 w315]
          tunnel: w273 -> [_ w300 w306 w314]
          tunnel: w272 -> [_ w299 w305 w313]
          tunnel: w271 -> [_ _ w304 w312]
          tunnel: w270 -> [_ _ w303 w311]
          tunnel: w269 -> [_ _ _ w310]
          tunnel: w268 -> [_ _ _ w309]
          frame "1", Default {
            "leftIndicator#1-1" <- w298
            "rightIndicator#1-1" <- w297
          }
          frame "2" {
            "leftIndicator#2-1" <- w302
            "rightIndicator#2-1" <- w300
            "leftIndicator#2-2" <- w301
            "rightIndicator#2-2" <- w299
          }
          frame "3" {
            "leftIndicator#3-1" <- w308
            "rightIndicator#3-1" <- w305
            "leftIndicator#3-3" <- w306
            "rightIndicator#3-3" <- w303
            "rightIndicator#3-2" <- w304
            "leftIndicator#3-2" <- w307
          }
          frame "4" {
            "leftIndicator#4-1" <- w316
            "rightIndicator#4-1" <- w312
            "leftIndicator#4-3" <- w314
            "rightIndicator#4-3" <- w310
            "rightIndicator#4-2" <- w311
            "leftIndicator#4-4" <- w313
            "rightIndicator#4-4" <- w309
            "leftIndicator#4-2" <- w315
          }
        }
      }
    }
    n145 = local read "Exit?"() -> (w263:bool)
    n146 = node-c288() -> ()  [unwired: 1 in, 1 out]
  }
  n147 = node-c288(w14) -> ()  [unwired: 1 out]
  n148 = disable-structure shown="비활성화" {
    disable-tunnel: w13 -> [w321 _]
    disable-tunnel: w12 -> [w320 _]
    disable-tunnel: w11 -> [w319 _]
    frame Disabled {
      n149 = stacked-sequence {
        tunnel: w321 -> [w322 _]
        tunnel: w320 -> [_ _]
        tunnel: w319 -> [_ _]
        frame #0 {
          # "마지막 설정 데이터를 DB에 저장"
          # "End Sequence #1"
          n150 = call "SerialCommunicationFGV.vi"("ctl"=T10."Close", "errorIn"=w322) -> ("VISA resource name out"=w323:refnum<visa-resource-name>)  [unwired: 7 in, 2 out]
          n151 = disable-structure shown="활성화" {
            frame Disabled {
              n152 = Bundle By Name(cluster=T3 {"Output High"=40.0, "Output Low"=-40.0, "Vel_FindBase"=5.0, "Ref.Load_FindBase"=5.0, "Force Peak"=0.0, "L_기준값"=81.0, "L_검출값"=103.0, "L_End%"=39.0, "L_Peak%"=25.0, "L_Onset%"=0.0, "L_Pos"=0.0, "L_Offset"=0.0, "R_기준값"=81.0, "R_검출값"=103.0, "R_End%"=39.0, "R_Peak%"=25.0, "R_Onset%"=0.0, "R_Pos"=0.0, "R_Offset"=0.0} ("Setting Value")) -> (w347:T3, "Output High"=w361:sgl, "Output Low"=w360:sgl, "Ref.Load_FindBase"=w359:sgl, "L_기준값"=w358:sgl, "L_End%"=w357:sgl, "L_Onset%"=w356:sgl, "L_Offset"=w355:sgl, "R_검출값"=w354:sgl, "R_Peak%"=w353:sgl, "R_Onset%"=w352:sgl, "R_Offset"=w351:sgl)  [unwired: 8 in]
              n153 = Cluster To Array(cluster=w347) -> (array=w346:sgl[])
              n154 = for {
                tunnel: w346 -> [w364] mode=indexing
                tunnel: [w363] -> w345 mode=indexing
                n155 = Number To Fractional String(number=w364) -> (F-format string=w363:string)  [unwired: 3 in]
              }
              n156 = Index Array(array=w345) -> (element #1=w344:string, element #2=w343:string, element #3=w342:string, element #4=w341:string, element #5=w340:string, element #6=w339:string, element #7=w338:string, element #8=w337:string, element #9=w336:string)  [unwired: 9 in]
              n157 = Format Into String(format string="INSERT INTO ROBOT_SETTING (\n    robot_setting_nm,\n    output_high,\n    output_low,\n    vel_find_base,\n    ref_load_find_base,\n    force_peak,\n    l_standard_value,\n    l_detected_value,\n    l_end_percent,\n    l_onset_percent,\n    l_peak_percent,\n    l_pos,\n    l_offset\n) VALUES (\n    '%s',  \n    %s,              -- output_high\n    %s,               -- output_low\n    %s,                -- vel_find_base\n    %s,               -- ref_load_find_base\n    %s,               -- force_peak\n    %s,                -- l_standard_value\n    %s,                -- l_detected_value\n    %s,               -- l_end_percent\n    %s,               -- l_onset_percent\n    %s,               -- l_peak_percent\n    %s,              -- l_pos\n    %s                 -- l_offset\n);\n", w344, w343, w342, w341, w340, w339, w338, w337, w336) -> (resulting string=w348:string)  [unwired: 3 in, 1 out]
              n158 = call "comDB.vi"("Query"=w348, "State"=T5."create") -> ()  [unwired: 5 in, 4 out]
            }
            frame Enabled {
            }
          }
          n159 = Bundle By Name(cluster=T6 {"baud rate (9600)"=9600, "flow control (0:none)"=0, "VISA resource name 2"="", "termination char\n(0xA = '\\n' = LF) "=10, "data bits (8)"=8, "parity (0:none)"=enum."None", "timeout (10sec)"=10000, "Enable Termination\nChar (T)"=TRUE, "stop bits (10: 1 bit)"=10} ("ViSA Config"), "VISA resource name 2"=w323, "baud rate (9600)"=u32 115200, "flow control (0:none)"=u16 0, "termination char\n(0xA = '\\n' = LF)"=u8 0 ("termination char\n(0xA = '\\n' = LF)"), "data bits (8)"=u16 8, "parity (0:none)"=enum16{"None", "Odd", "Even", "Mark", "Space"}."None", "timeout (10sec)"=u32 10, "Enable Termination\nChar (T)"=FALSE ("Enable Termination\nChar (T)"), "stop bits (10: 1 bit)"=u16 0) -> (w326:T6)
          n160 = call "serialConfigSave.vi"("Ctl"=enum16{"read", "write"}."write", "ViSA Config"=w326) -> ()  [unwired: 9 in, 1 out]
        }
        frame #1 {
          # "해당 VI 종료 (참조 닫기 등...)"
          # "End Sequence #1"
          n161 = call "PannelControl.vi"("State"=T11."Home") -> ()  [unwired: 10 in, 1 out]
        }
      }
    }
    frame Enabled {
    }
  }
  n162 = RT FIFO Delete(0:w1, 3:w2) -> ()  [unwired: 1 in, 1 out]
